vi "Get LabVIEW Install Paths.vi"(8 "Error In":errorcluster) -> (0 "Error Out":errorcluster, 2 "LV Directories":path[](array[path]), 3 "LV Version":string[](array[string]))   [LabVIEW 2011, in "LVH-Toolbox.lvlib" / "LVH-Common.lvlib"]
uses:
  <vilib>/registry/registry.llb/Read Registry Value Simple STR.vi
  LVH-Common.lvlib
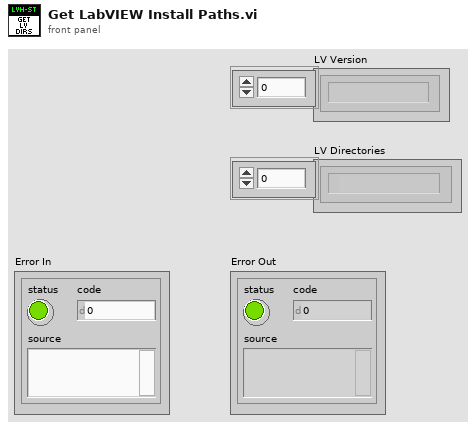
[diagram p1: front panel]
types:
  T1 = typedef "Registry refnum.ctl" = refnum<k1>
  T2 = cluster{"numSubKeys":i32, "maxSubKeyLen":i32, "maxSubKeyClassLen":i32}
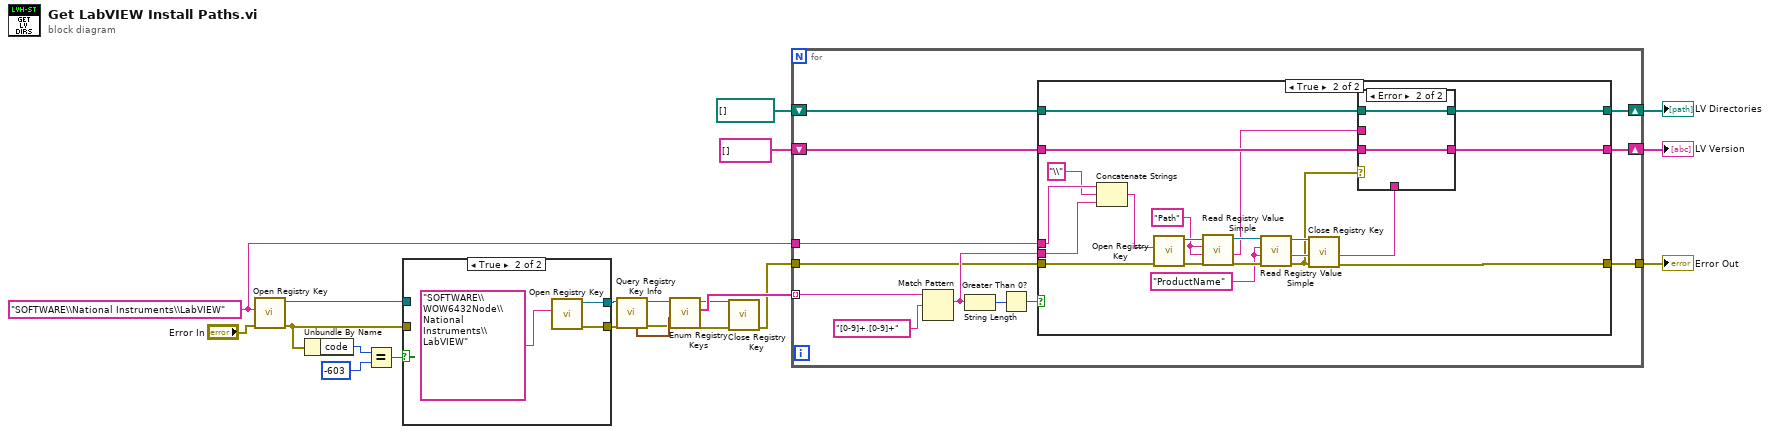
[diagram p0: block diagram]
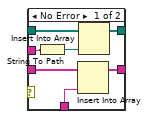
[diagram p4: hidden frame]
diagram:
  w15 = "SOFTWARE\\National Instruments\\LabVIEW" ("subkey")
  n1 = call <vilib>:"Open Registry Key.vi"("error in (no error)"="Error In", "subkey"=w15) -> ("error out"=w4:errorcluster, "refnum out"=w2:T1)  [unwired: 8 in]
  n2 = Unbundle By Name(w4) -> ("code"=w7:i32)
  n3 = Equal?(x=w7, y=-603) -> (x = y?=w5:bool)
  n4 = case shown="True" w5 {
    tunnel: w4 -> [w22 _]
    tunnel: [w23 w25] -> w3
    tunnel: w2 -> [w23 _]
    tunnel: [w22 w24] -> w1
    frame False {
      # "Found x32 Entry"
    }
    frame True {
      n5 = call <vilib>:"Open Registry Key.vi"("subkey"="SOFTWARE\\WOW6432Node\\National Instruments\\LabVIEW") -> ("error out"=w24:errorcluster, "refnum out"=w25:T1)  [unwired: 9 in]
    }
  }
  n6 = call <vilib>:"Query Registry Key Info.vi"("error in (no error)"=w1, "refnum"=w3) -> ("error out"=w19:errorcluster, "refnum out"=w21:T1, "subkey info"=w20:T2)  [unwired: 5 in, 2 out]
  n7 = call <vilib>:"Enum Registry Keys.vi"("error in (no error)"=w19, "subkey info"=w20, "refnum"=w21) -> ("error out"=w16:errorcluster, "subkeys"=w18:string[], "refnum out"=w17:T1)  [unwired: 6 in]
  n8 = call <vilib>:"Close Registry Key.vi"("error in (no error)"=w16, "refnum"=w17) -> ("error out"=w14:errorcluster)  [unwired: 5 in]
  n9 = for {
    tunnel: w18 -> [w38] mode=indexing
    tunnel: w15 -> [w34]
    shift-right: [w29] -> w10
    shift-left: string[] [] -> [w30]
    shift-right: [w27] -> w8
    shift-left: path[] [] -> [w28]
    tunnel: w14 -> [w32]
    tunnel: [w31] -> w12
    n10 = Match Pattern(string=w38, regular expression="[0-9]+.[0-9]+") -> (match substring=w33:string)  [unwired: 1 in, 3 out]
    n11 = String Length(string=w33) -> (length=w36:i32)
    n12 = Greater Than 0?(x=w36) -> (x > 0?=w35:bool)
    n13 = case shown="True" w35 {
      tunnel: w34 -> [_ w61]
      tunnel: w33 -> [_ w57]
      tunnel: w32 -> [w41 w59]
      tunnel: [w41 w53] -> w31
      tunnel: w30 -> [w39 w48]
      tunnel: [w39 w46] -> w29
      tunnel: w28 -> [w40 w45]
      tunnel: [w40 w44] -> w27
      frame False {
      }
      frame True {
        w49 = "ProductName" ("value")
        w54 = "Path" ("value")
        n14 = Concatenate Strings(w61, "\\" ("string"), w57) -> (w60:string)
        n15 = call <vilib>:"Open Registry Key.vi"("error in (no error)"=w59, "subkey"=w60) -> ("error out"=w55:errorcluster, "refnum out"=w56:T1)  [unwired: 8 in]
        n16 = call-poly <vilib>:"Read Registry Value Simple.vi"("error in (no error)"=w55, "default data"=w54, "value"=w54, "refnum"=w56) -> ("error out"=w52:errorcluster, "String/Binary data"=w43:string, "refnum out"=w51:T1)  [unwired: 2 in, 1 out]
        n17 = call-poly <vilib>:"Read Registry Value Simple.vi"("error in (no error)"=w52, "default data"=w49, "value"=w49, "refnum"=w51) -> ("error out"=w42:errorcluster, "String/Binary data"=w47:string, "refnum out"=w50:T1)  [unwired: 2 in, 1 out]
        n18 = call <vilib>:"Close Registry Key.vi"("error in (no error)"=w42, "refnum"=w50) -> ("error out"=w53:errorcluster)  [unwired: 5 in]
        n19 = case shown="Error" w42 {
          tunnel: w48 -> [w68 w69]
          tunnel: w47 -> [w67 _]
          tunnel: [w66 w69] -> w46
          tunnel: w45 -> [w65 w70]
          tunnel: [w64 w70] -> w44
          tunnel: w43 -> [w63 _]
          frame No Error {
            n20 = String To Path(string=w63) -> (path=w62:path)
            n21 = Insert Into Array(array=w68, new element=w67) -> (w66:string[])  [unwired: 1 in]
            n22 = Insert Into Array(array=w65, new element=w62) -> (w64:path[])  [unwired: 1 in]
          }
          frame Error {
          }
        }
      }
    }
  }
  "Error Out" <- w12
  "LV Version" <- w10
  "LV Directories" <- w8
